vi "Lowpass Image.vi"(8 "error in":errorcluster, 10 "Lowpass IN":T2, 11 "Refnum in":T1) -> (0 "error out":errorcluster, 3 "Refnum out":T1)   [LabVIEW 2020]
uses:
  <vilib>/vision/Image Controls.llb/IMAQ Image.ctl
  <vilib>/vision/NI_Vision_Development_Module.lvlib
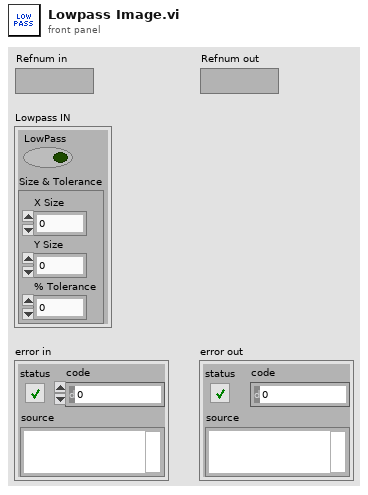
[diagram p1: front panel]
types:
  T1 = typedef "IMAQ Image.ctl" = refnum<image>
  T2 = cluster{"LowPass":bool, "Size & Tolerance":cluster{"X Size":i32, "Y Size":i32, "% Tolerance":i32}}
  T3 = cluster{"X Size":i32, "Y Size":i32, "% Tolerance":i32}
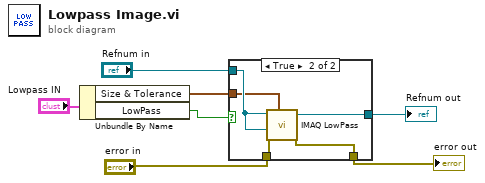
[diagram p0: block diagram]
diagram:
  n1 = Unbundle By Name("Lowpass IN") -> ("Size & Tolerance"=w2:T3, "LowPass"=w1:bool)
  n2 = case shown="True" w1 {
    tunnel: "Refnum in" -> [w9 w13]
    tunnel: [w9 w14] -> w5
    tunnel: "error in" -> [w8 w12]
    tunnel: [w8 w10] -> w7
    tunnel: w2 -> [_ w11]
    frame False {
    }
    frame True {
      n3 = call "IMAQ LowPass"("Image Src"=w13, "Size & Tolerance"=w11, "Image Dst"=w13, "error in (no error)"=w12) -> ("Image Dst Out"=w14:T1, "error out"=w10:errorcluster)  [unwired: 3 in]
    }
  }
  "error out" <- w7
  "Refnum out" <- w5
